vi "X-ray-images-mergening and calculating.vi"() -> ()   [LabVIEW 2019]
uses:
  <vilib>/Utility/file.llb/Write Delimited Spreadsheet (string).vi
  <vilib>/vision/NI_Vision_Development_Module.lvlib
  <vilib>/gmath/NI_Gmath.lvlib
  <vilib>/Analysis/NI_AALBase.lvlib
  imFillRemove_vs2019/x64/Release/imFillRemove_vs2019.dll
  distance_VS2019/x64/Release/distance_VS2019.dll
panel:
  out "Boolean":bool
  out "Path(part1)":path
  out "Path(part2)":path
  out "the lastest":string
  out "点击次数：":i32
  out "standard deviation 9":dbl format="%0.2f"
  out "mean 9":dbl format="%0.2f"
  out "standard deviation 8":dbl format="%0.2f"
  out "mean 8":dbl format="%0.2f"
  out "standard deviation 7":dbl format="%0.2f"
  out "mean 7":dbl format="%0.2f"
  out "standard deviation 6":dbl format="%0.2f"
  out "mean 6":dbl format="%0.2f"
  out "standard deviation 5":dbl format="%0.2f"
  out "mean 5":dbl format="%0.2f"
  out "Circularity":dbl[](array[numeric])
  out "Equivalent ellipse":dbl[](array[numeric])
  out "AR":dbl[](array[numeric])
  out "Perimeter":dbl[](array[numeric])
  out "Area":dbl[](array[numeric])
  out "耗时":u32
  out "属于某个角度下图像":T1(plugin-control)
  out "粒长":dbl[](array[numeric])
  out "粒宽":dbl[](array[numeric])
  out "长宽比":dbl[](array[numeric])
  out "mean 2":dbl format="%0.2f"
  out "standard deviation 2":dbl format="%0.2f"
  out "mean 3":dbl format="%0.2f"
  out "standard deviation 3":dbl format="%0.2f"
  out "mean 4":dbl format="%0.2f"
  out "standard deviation 4":dbl format="%0.2f"
  out "Number of Particles 2":i32
  out "单个粒子":T1(plugin-control)
  out "Combine Image final label 2":T1(plugin-control)
  in  "Removeareathreshold":i32=100
  in  "Range 2":cluster{"Lower value":sgl, "Upper value":sgl}={"Lower value"=1.0, "Upper value"=120.0}
  in  "数据存储":path=path "G:/preprocessing/rice_panicle/CT/data.xls"
  out "mean value 2":dbl
  in  "图片存储":path=path "G:/preprocessing/rice_panicle/CT/CT-merge"
  out "Combine Image":T1(plugin-control)
  out "Current Click Point":i32[](array[numeric])
  in  "CT images combine Stop":bool
  out "Click Points Array 2":i32[][](array[numeric])
  out "Combine Image final":T1(plugin-control)
  out "Combine Image final label":T1(plugin-control)
  out "Combine Image final label diatance":T1(plugin-control)
  out "Solid particle number（自动测量）":i32
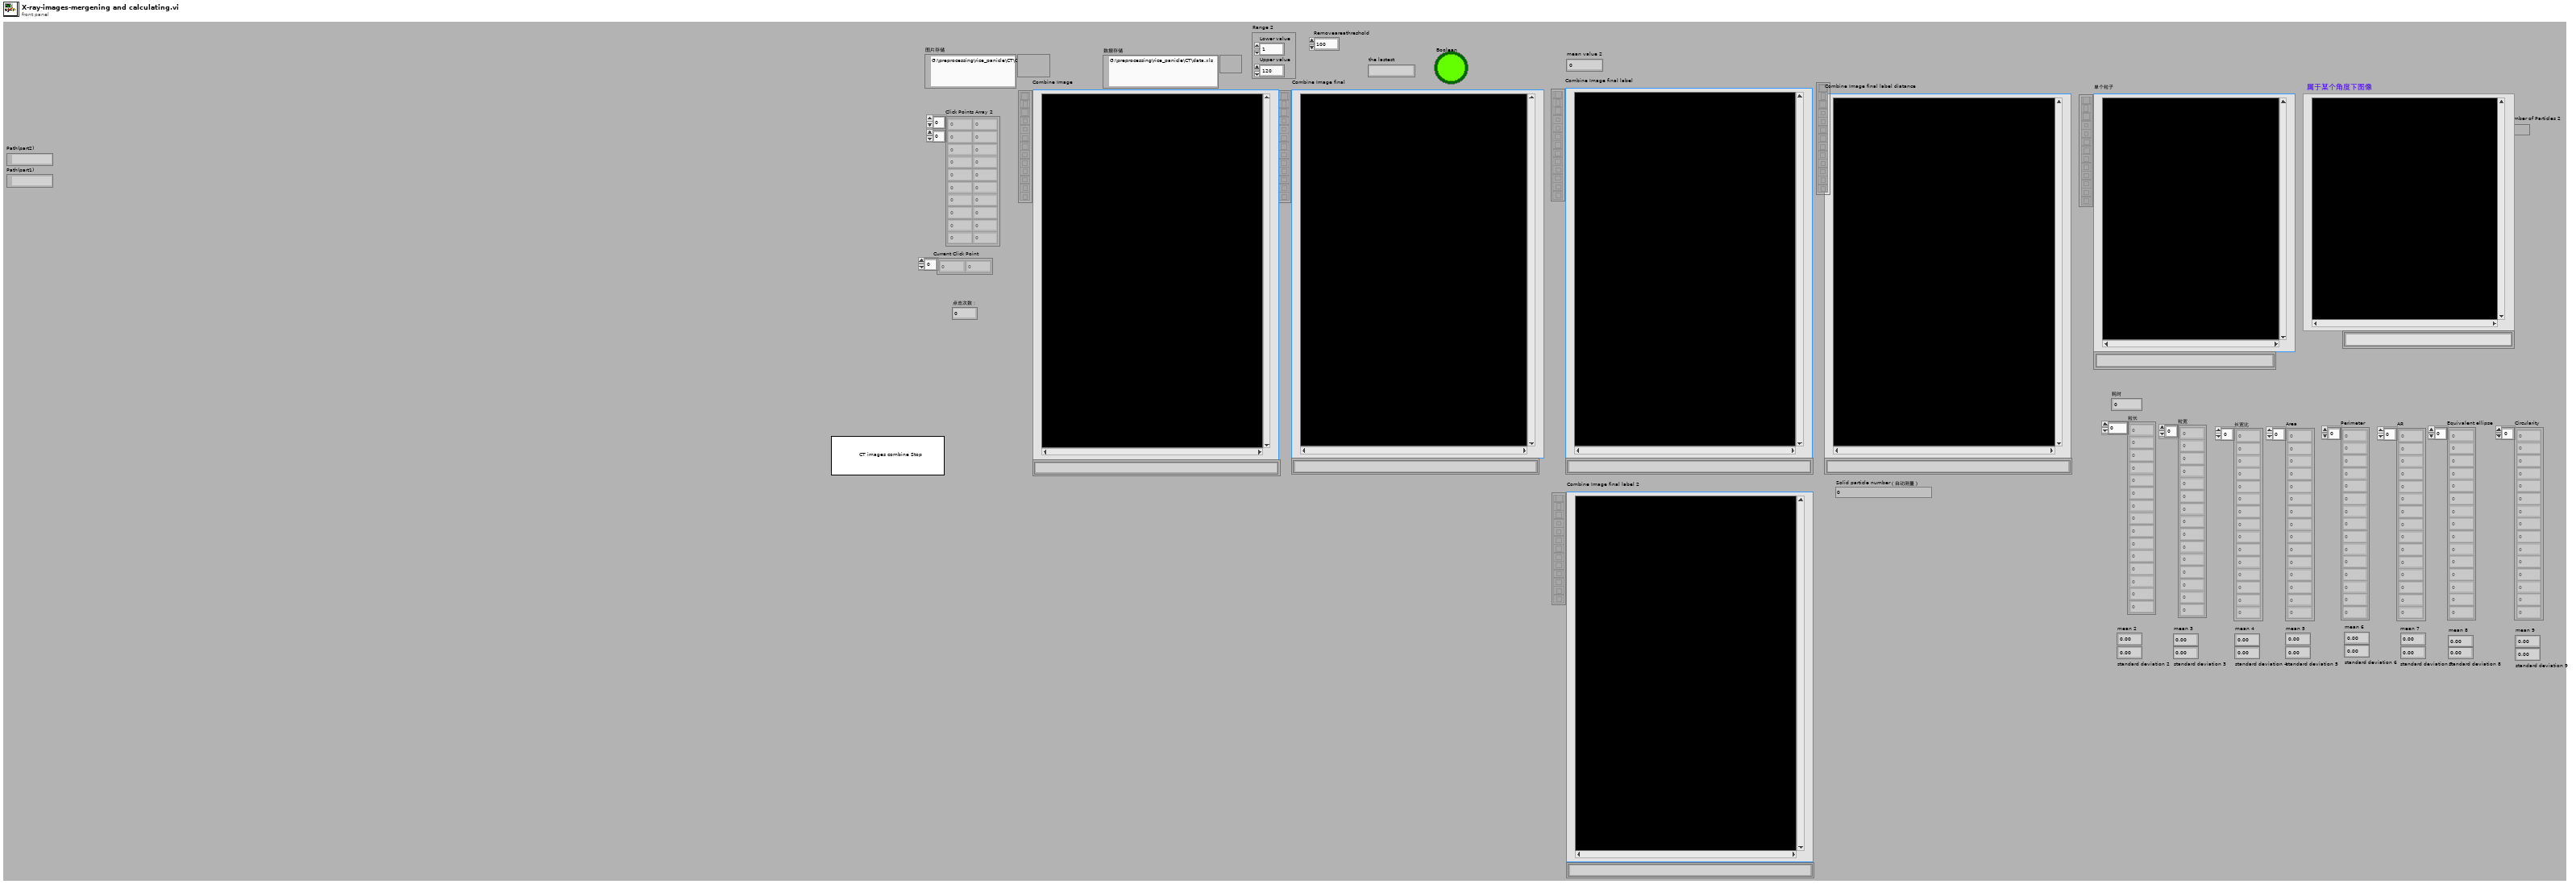
[diagram p1: front panel]
types:
  T1 = typedef "IMAQ Image.ctl" = refnum<image>
  T2 = typedef "Particle Parameters" = i32
  T3 = cluster{"Measurement Parameter":T2, "Range Lower Value":dbl, "Range Upper Value":dbl, "Range":bool, "Measurement Type":bool}
  T4 = enum16{"arithmetic", "geometric", "harmonic", "trimmed", "median"}
  T5 = typedef "Image Type" = u32
  T6 = cluster{"Measurement Parameter":T2, "Range Lower Value":dbl, "Range Upper Value":dbl, "Range":bool, "Measurement Type":bool}[]
  T7 = cluster{"Measurement Parameter":T2, dbl, dbl, "Range":bool, "Measurement Type":bool}
  T8 = cluster{"Measurement Parameter":T2, dbl, dbl, "Range":bool, "Measurement Type":bool}[]
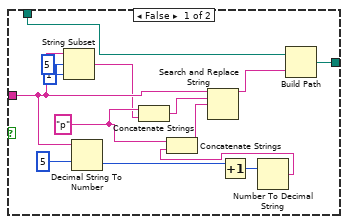
[diagram p2: hidden frame]
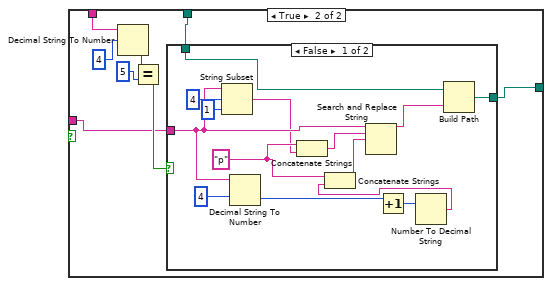
[diagram p3: hidden frame]
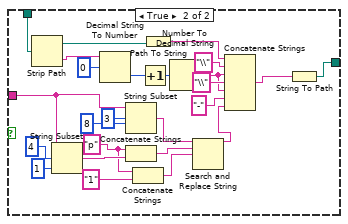
[diagram p4: hidden frame]
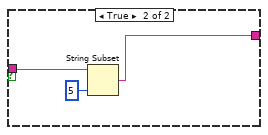
[diagram p5: hidden frame]
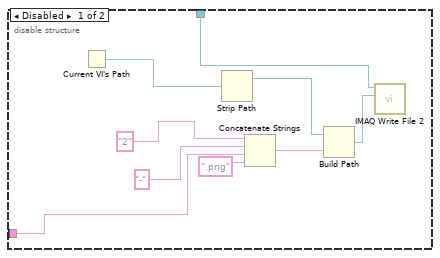
[diagram p6: hidden frame]
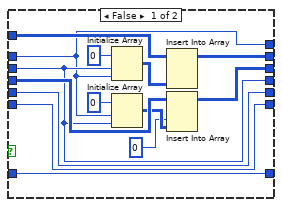
[diagram p8: hidden frame]
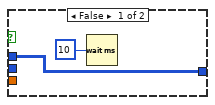
[diagram p9: hidden frame]
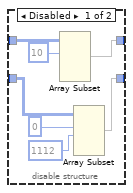
[diagram p10: hidden frame]
diagram:
  n1 = flat-sequence {
    tunnel: [w3] -> w2
    tunnel: [w5] -> w1
    frame #0 {
      n2 = call "IMAQ Load Image Dialog"("Prompt"="Select a panicle ct image (part1)") -> ("Path"=w3:path)  [unwired: 6 in, 4 out]
    }
    frame #1 {
      n3 = call "IMAQ Load Image Dialog"("Prompt"="Select a panicle ct image (part2)") -> ("Path"=w5:path)  [unwired: 6 in, 4 out]
    }
  }
  n4 = while {
    shift-right: [w12] -> _
    shift-left: w1 -> [w24]
    shift-right: [w11] -> _
    shift-left: w2 -> [w16]
    stop <- FALSE stop-if-true
    n5 = Strip Path(path=w16) -> (name=w18:string)  [unwired: 1 out]
    n6 = String Subset(string=w18, offset (0)=2, length (rest)=1 ("length (rest)")) -> (substring=w21:string)
    n7 = Equal?(x=w21, y="-") -> (x = y?=w19:bool)
    n8 = case shown="False" w19 {
      tunnel: w18 -> [w130 w133]
      tunnel: [w129 w132] -> w17
      frame False {
        n9 = String Subset(string=w130, length (rest)=6 ("length (rest)")) -> (substring=w129:string)  [unwired: 1 in]
      }
      frame True {
        n10 = String Subset(string=w133, length (rest)=5 ("length (rest)")) -> (substring=w132:string)  [unwired: 1 in]
      }
    }
    "the lastest" <- w17
    n11 = flat-sequence {
      tunnel: w16 -> [w136]
      tunnel: w24 -> [w135]
      frame #0 {
        w169 = T2[] [35, 19, 32, 50, 55] items=["Center of Mass X", "Center of Mass Y", "First Pixel X", "First Pixel Y", "Bounding Rect Left", "Bounding Rect Top", "Bounding Rect Right", "Bounding Rect Bottom", "Max Feret Diameter Start X", "Max Feret Diameter Start Y", "Max Feret Diameter End X", "Max Feret Diameter End Y", "Max Horiz. Segment Length Left", "Max Horiz. Segment Length Right", "Max Horiz. Segment Length Row", "-", "Bounding Rect Width", "Bounding Rect Height", "Bounding Rect Diagonal", "Perimeter", "Convex Hull Perimeter", "Holes' Perimeter", "Max Feret Diameter", "Equivalent Ellipse Major Axis", "Equivalent Ellipse Minor Axis", "Equivalent Ellipse Minor Axis (Feret)", "Equivalent Rect Long Side", "Equivalent Rect Short Side", "Equivalent Rect Diagonal", "Equivalent Rect Short Side (Feret)", "Average Horiz. Segment Length", "Average Vert. Segment Length", "Hydraulic Radius", "Waddel Disk Diameter", "-", "Area", "Holes' Area", "Particle & Holes' Area", "Convex Hull Area", "Image Area", "-", "Number of Holes", "Number of Horiz. Segments", "Number of Vert. Segments", "-", "Orientation", "Max Feret Diameter Orientation", "-", "% Area/Image Area", "% Area/(Particle & Holes' Area)", "Ratio of Equivalent Ellipse Axes", "Ratio of Equivalent Rect Sides", "-", "Elongation Factor", "Compactness Factor", "Heywood Circularity Factor", "Type Factor", "-", "Sum X", "Sum Y", "Sum XX", "Sum XY", "Sum YY", "Sum XXX", "Sum XXY", "Sum XYY", "Sum YYY", "-", "Moment of Inertia XX", "Moment of Inertia XY", "Moment of Inertia YY", "Moment of Inertia XXX", "Moment of Inertia XXY", "Moment of Inertia XYY", "Moment of Inertia YYY", "Norm. Moment of Inertia XX", "Norm. Moment of Inertia XY", "Norm. Moment of Inertia YY", "Norm. Moment of Inertia XXX", "Norm. Moment of Inertia XXY", "Norm. Moment of Inertia XYY", "Norm. Moment of Inertia YYY", "Hu Moment 1", "Hu Moment 2", "Hu Moment 3", "Hu Moment 4", "Hu Moment 5", "Hu Moment 6", "Hu Moment 7"] ("Pixel Measurements")
        w177 = T2[] [35] items=["Center of Mass X", "Center of Mass Y", "First Pixel X", "First Pixel Y", "Bounding Rect Left", "Bounding Rect Top", "Bounding Rect Right", "Bounding Rect Bottom", "Max Feret Diameter Start X", "Max Feret Diameter Start Y", "Max Feret Diameter End X", "Max Feret Diameter End Y", "Max Horiz. Segment Length Left", "Max Horiz. Segment Length Right", "Max Horiz. Segment Length Row", "-", "Bounding Rect Width", "Bounding Rect Height", "Bounding Rect Diagonal", "Perimeter", "Convex Hull Perimeter", "Holes' Perimeter", "Max Feret Diameter", "Equivalent Ellipse Major Axis", "Equivalent Ellipse Minor Axis", "Equivalent Ellipse Minor Axis (Feret)", "Equivalent Rect Long Side", "Equivalent Rect Short Side", "Equivalent Rect Diagonal", "Equivalent Rect Short Side (Feret)", "Average Horiz. Segment Length", "Average Vert. Segment Length", "Hydraulic Radius", "Waddel Disk Diameter", "-", "Area", "Holes' Area", "Particle & Holes' Area", "Convex Hull Area", "Image Area", "-", "Number of Holes", "Number of Horiz. Segments", "Number of Vert. Segments", "-", "Orientation", "Max Feret Diameter Orientation", "-", "% Area/Image Area", "% Area/(Particle & Holes' Area)", "Ratio of Equivalent Ellipse Axes", "Ratio of Equivalent Rect Sides", "-", "Elongation Factor", "Compactness Factor", "Heywood Circularity Factor", "Type Factor", "-", "Sum X", "Sum Y", "Sum XX", "Sum XY", "Sum YY", "Sum XXX", "Sum XXY", "Sum XYY", "Sum YYY", "-", "Moment of Inertia XX", "Moment of Inertia XY", "Moment of Inertia YY", "Moment of Inertia XXX", "Moment of Inertia XXY", "Moment of Inertia XYY", "Moment of Inertia YYY", "Norm. Moment of Inertia XX", "Norm. Moment of Inertia XY", "Norm. Moment of Inertia YY", "Norm. Moment of Inertia XXX", "Norm. Moment of Inertia XXY", "Norm. Moment of Inertia XYY", "Norm. Moment of Inertia YYY", "Hu Moment 1", "Hu Moment 2", "Hu Moment 3", "Hu Moment 4", "Hu Moment 5", "Hu Moment 6", "Hu Moment 7"] ("Pixel Measurements")
        w179 = T5 0 items=["Grayscale (U8)", "Grayscale (I16)", "Grayscale (SGL)", "Complex (CSG)", "RGB (U32)", "HSL (U32)", "RGB (U64)", "Grayscale (U16)"] ("Image Type")
        n12 = while {
          tunnel: [w435] -> _
          tunnel: [w434] -> w234
          tunnel: [w433] -> w232
          tunnel: [w432] -> w222
          tunnel: [w431] -> w221
          tunnel: w135 -> [w430]
          tunnel: [w429] -> w213
          tunnel: [w428] -> w207
          tunnel: [w419] -> w210
          tunnel: w136 -> [w418]
          stop <- w420 stop-if-true
          n13 = flat-sequence {
            tunnel: w430 -> [w444]
            tunnel: w418 -> [w446]
            tunnel: [w467] -> w427
            tunnel: [w464] -> w426
            tunnel: [w459] -> w425
            tunnel: [w456] -> w424
            tunnel: [w453] -> w423
            tunnel: [w445] -> w422
            tunnel: [w437] -> w421
            tunnel: [w444] -> w419
            tunnel: [w610] -> w428
            tunnel: [w611] -> w429
            tunnel: [w612] -> w431
            tunnel: [w613] -> w432
            tunnel: [w614] -> w433
            tunnel: [w615] -> w434
            tunnel: [w616] -> w435
            tunnel: w427 -> [w616]
            tunnel: w426 -> [w615]
            tunnel: w425 -> [w614]
            tunnel: w424 -> [w613]
            tunnel: w423 -> [w612]
            tunnel: w422 -> [w611]
            tunnel: w421 -> [w610]
            tunnel: [w609] -> w420
            frame #0 {
              w454 = u32 0 items=["Grayscale (U8)", "Grayscale (I16)", "Grayscale (SGL)", "Complex (CSG)", "RGB (U32)", "HSL (U32)", "RGB (U64)"] ("Image Type")
              w457 = u32 0 items=["Grayscale (U8)", "Grayscale (I16)", "Grayscale (SGL)", "Complex (CSG)", "RGB (U32)", "HSL (U32)", "RGB (U64)"] ("Image Type")
              w460 = u32 0 items=["Grayscale (U8)", "Grayscale (I16)", "Grayscale (SGL)", "Complex (CSG)", "RGB (U32)", "HSL (U32)", "RGB (U64)"] ("Image Type")
              w462 = u32 0 items=["Grayscale (U8)", "Grayscale (I16)", "Grayscale (SGL)", "Complex (CSG)", "RGB (U32)", "HSL (U32)", "RGB (U64)"] ("Image Type")
              w465 = u32 0 items=["Grayscale (U8)", "Grayscale (I16)", "Grayscale (SGL)", "Complex (CSG)", "RGB (U32)", "HSL (U32)", "RGB (U64)"] ("Image Type")
              w468 = u32 0 items=["Grayscale (U8)", "Grayscale (I16)", "Grayscale (SGL)", "Complex (CSG)", "RGB (U32)", "HSL (U32)", "RGB (U64)"] ("Image Type")
              w484 = u32 0 items=["Grayscale (U8)", "Grayscale (I16)", "Grayscale (SGL)", "Complex (CSG)", "RGB (U32)", "HSL (U32)", "RGB (U64)"] ("Image Type")
              w517 = i32[] [1] items=["No  event", "Click event", "Draw event", "Move event", "Size event", "Scroll event", "Activate event", "Close event", "Double click event"] ("Events list (all)")
              w528 = T5 0 items=["Grayscale (U8)", "Grayscale (I16)", "Grayscale (SGL)", "Complex (CSG)", "RGB (U32)", "HSL (U32)", "RGB (U64)", "Grayscale (U16)"] ("Image Type")
              w530 = T5 0 items=["Grayscale (U8)", "Grayscale (I16)", "Grayscale (SGL)", "Complex (CSG)", "RGB (U32)", "HSL (U32)", "RGB (U64)", "Grayscale (U16)"] ("Image Type")
              w537 = u32 0 items=["Grayscale (U8)", "Grayscale (I16)", "Grayscale (SGL)", "Complex (CSG)", "RGB (U32)", "HSL (U32)", "RGB (U64)"] ("Image Type")
              w540 = T5 0 items=["Grayscale (U8)", "Grayscale (I16)", "Grayscale (SGL)", "Complex (CSG)", "RGB (U32)", "HSL (U32)", "RGB (U64)", "Grayscale (U16)"] ("Image Type")
              w543 = T5 0 items=["Grayscale (U8)", "Grayscale (I16)", "Grayscale (SGL)", "Complex (CSG)", "RGB (U32)", "HSL (U32)", "RGB (U64)", "Grayscale (U16)"] ("Image Type")
              n14 = call "IMAQ Create"("Image Name"="part2", "Image Type"=w540) -> ("New Image"=w542:T1)  [unwired: 2 in, 2 out]
              n15 = call "IMAQ Create"("Image Name"="distance2_ct", "Image Type"=w457) -> ("New Image"=w456:T1)  [unwired: 2 in, 2 out]
              n16 = call "IMAQ Create"("Image Name"="part1", "Image Type"=w543) -> ("New Image"=w545:T1)  [unwired: 2 in, 2 out]
              n17 = call "IMAQ Create"("Image Name"="combine_final", "Image Type"=w484) -> ("New Image"=w483:T1)  [unwired: 2 in, 2 out]
              n18 = call "IMAQ Create"("Image Name"="part2 rotate", "Image Type"=w528) -> ("New Image"=w524:T1)  [unwired: 2 in, 2 out]
              n19 = call "IMAQ Create"("Image Name"="part1 rotate", "Image Type"=w530) -> ("New Image"=w526:T1)  [unwired: 2 in, 2 out]
              n20 = call "IMAQ Create"("Image Name"="combine", "Image Type"=w537) -> ("New Image"=w536:T1)  [unwired: 2 in, 2 out]
              n21 = call "IMAQ Create"("Image Name"="cluster_ct", "Image Type"=w462) -> ("New Image"=w445:T1)  [unwired: 2 in, 2 out]
              n22 = call "IMAQ Create"("Image Name"="threshold_ct", "Image Type"=w468) -> ("New Image"=w467:T1)  [unwired: 2 in, 2 out]
              n23 = call "IMAQ Create"("Image Name"="labelImage_ct", "Image Type"=w465) -> ("New Image"=w464:T1)  [unwired: 2 in, 2 out]
              n24 = call "IMAQ Create"("Image Name"="diatance_ct", "Image Type"=w460) -> ("New Image"=w459:T1)  [unwired: 2 in, 2 out]
              n25 = call "IMAQ Create"("Image Name"="labelImage3_ct", "Image Type"=w454) -> ("New Image"=w453:T1)  [unwired: 2 in, 2 out]
              n26 = call "IMAQ ReadFile"("File Path"=w444, "Image"=w542) -> ("Image Out"=w523:T1)  [unwired: 3 in, 6 out]
              n27 = call "IMAQ ReadFile"("File Path"=w446, "Image"=w545) -> ("Image Out"=w525:T1)  [unwired: 3 in, 6 out]
              n28 = call "IMAQ Rotate"("Maintain Size"=FALSE, "Angle (degrees)"=sgl 90.0, "Image Dst"=w524, "Image Src"=w523) -> ("Image Dst Out"=w531:T1)  [unwired: 4 in, 3 out]
              n29 = call "IMAQ Rotate"("Maintain Size"=FALSE, "Angle (degrees)"=sgl 90.0, "Image Dst"=w526, "Image Src"=w525) -> ("Image Dst Out"=w522:T1)  [unwired: 4 in, 3 out]
              n30 = call "IMAQ ImageToArray"("Image"=w531) -> ("Image Pixels (U8)"=w514:u8[][])  [unwired: 2 in, 5 out]
              n31 = call "IMAQ ImageToArray"("Image"=w522) -> ("Image Pixels (U8)"=w515:u8[][])  [unwired: 2 in, 5 out]
              n32 = disable-structure shown="Enabled" {
                disable-tunnel: w514 -> [w606 w607]
                disable-tunnel: w515 -> [w604 w608]
                disable-tunnel: [w601 w608] -> w521
                disable-tunnel: [w600 w607] -> w520
                frame Disabled {
                  n33 = Array Subset(array=w606, index (row)=10 ("index")) -> (w600:u8[][])  [unwired: 3 in]
                  n34 = Array Subset(array=w604, index (row)=0 ("index"), length (row)=1112 ("length")) -> (w601:u8[][])  [unwired: 2 in]
                }
                frame Enabled {
                }
              }
              n35 = Insert Into Array(array=w521, new element=w520) -> (w539:u8[][])  [unwired: 2 in]
              n36 = call "IMAQ ArrayToImage"("Image Pixels (U8)"=w539, "Image"=w536) -> ("Image Out"=w516:T1)  [unwired: 4 in, 5 out]
              "Combine Image" <- w516
              n37 = invoke on="Combine Image" class="ImageControl" method="Clear ROI"() -> (error out=w518:errorcluster)  [unwired: 3 in, 2 out]
              n38 = while {
                tunnel: w517 -> [w593]
                tunnel: w518 -> [_]
                shift-right: [w584] -> w506
                shift-left: i32[][] [] ("appended array") -> [w589]
                tunnel: w516 -> [_]
                tunnel: w515 -> [w588]
                tunnel: w514 -> [w587]
                tunnel: [w588] -> w500
                tunnel: [w587] -> w499
                stop <- w585 stop-if-true
                n39 = invoke on="Combine Image" class="ImageControl" method="Get Last Event"("Which Events"=w593) -> ("Type"=w592:i32, "Coordinates"=w591:i32[], "Other Parameters"=w590:sgl[])  [unwired: 7 in, 5 out]
                n40 = Not Equal To 0?(x=w592) -> (x != 0?=w594:bool)
                n41 = case shown="True" w594 {
                  tunnel: w591 -> [_ w598]
                  tunnel: w590 -> [_ _]
                  tunnel: w589 -> [w595 w599]
                  tunnel: [w595 w597] -> w584
                  frame False {
                    n42 = Wait (ms)(milliseconds to wait=u32 10) -> ()  [unwired: 1 out]
                  }
                  frame True {
                    n43 = Build Array (concatenate)(w599, w598) -> (w597:i32[][])
                    "Current Click Point" <- w598
                  }
                }
                n44 = Index Array(array=w584, index (col)=0 ("disabled index (col)")) -> (element=w582:i32[])  [unwired: 1 in]
                n45 = Array Size(array=w582) -> (size(s)=w581:i32)
                "点击次数：" <- w581
                n46 = Equal?(x=w581, y=2) -> (x = y?=w585:bool)
              }
              "Click Points Array 2" <- w506
              n47 = Array Size(array=w500) -> (size(s)=w496:i32[])
              n48 = Index Array(array=w506, index (row)=0) -> (element=w508:i32[])  [unwired: 1 in]
              n49 = Index Array(array=w506, index (row)=1) -> (element=w489:i32[])  [unwired: 1 in]
              n50 = Index Array(array=w496, index=1) -> (element=w494:i32)
              n51 = Index Array(array=w496, index=0) -> (element=w495:i32)
              n52 = Index Array(array=w508, index=1) -> (element=w498:i32)
              n53 = Index Array(array=w508, index=0) -> (element=w504:i32)
              n54 = Index Array(array=w489, index=0) -> (element=w503:i32)
              n55 = Index Array(array=w489, index=1) -> (element=w488:i32)
              n56 = Subtract(x=w504, y=w503) -> (x-y=w481:i32)
              n57 = Absolute Value(x=w481) -> (abs(x)=w482:i32)
              n58 = Greater Or Equal?(x=w481, y=0) -> (x >= y?=w501:bool)
              n59 = case shown="True" w501 {
                tunnel: w500 -> [w559 w568]
                tunnel: w499 -> [w556 w573]
                tunnel: w498 -> [w562 w577]
                tunnel: w495 -> [w563 w576]
                tunnel: w494 -> [w553 w570]
                tunnel: w482 -> [w554 w569]
                tunnel: [w560 w567] -> w493
                tunnel: [w555 w574] -> w492
                tunnel: [w562 w577] -> w491
                tunnel: [w563 w576] -> w478
                tunnel: w488 -> [w561 w575]
                tunnel: [w561 w575] -> w480
                tunnel: [w553 w570] -> _
                tunnel: [w554 w569] -> w476
                frame False {
                  n60 = Initialize Array(u8 0 ("element"), w554, w553) -> (w565:u8[][])
                  n61 = Initialize Array(u8 0 ("element"), w553, w554) -> (w558:u8[][])
                  n62 = Insert Into Array(array=w556, new element=w565) -> (w555:u8[][])  [unwired: 2 in]
                  n63 = Insert Into Array(array=w559, index (col)=0 ("disabled index (col)"), new element=w558) -> (w560:u8[][])  [unwired: 1 in]
                }
                frame True {
                  n64 = Initialize Array(u8 0 ("element"), w570, w569) -> (w571:u8[][])
                  n65 = Initialize Array(u8 0 ("element"), w570, w569) -> (w579:u8[][])
                  n66 = Insert Into Array(array=w573, index (col)=0 ("disabled index (col)"), new element=w571) -> (w574:u8[][])  [unwired: 1 in]
                  n67 = Insert Into Array(array=w568, new element=w579) -> (w567:u8[][])  [unwired: 2 in]
                }
              }
              n68 = Subtract(x=w480, y=w478) -> (x-y=w479:i32)
              n69 = Array Subset(array=w493, index (row)=0 ("index"), length (row)=w491) -> (w487:u8[][])  [unwired: 2 in]
              n70 = Add(x=w476, y=10) -> (x+y=w475:i32)
              n71 = Array Subset(array=w492, index (row)=w479) -> (w486:u8[][])  [unwired: 3 in]
              n72 = Insert Into Array(array=w487, new element=w486) -> (w473:u8[][])  [unwired: 2 in]
              n73 = Array Subset(array=w473, index (row)=10 ("index"), length (row)=2600 ("length"), index (col)=w475, length (col)=1850 ("length")) -> (w470:u8[][])
              n74 = call "IMAQ ArrayToImage"("Image Pixels (U8)"=w470, "Image"=w483) -> ("Image Out"=w447:T1)  [unwired: 4 in, 5 out]
              n75 = call "IMAQ ImageBorderSize"("Get/Set Status? (Set)"=TRUE, "Image"=w447, "Image border size in"=5 ("Border Size")) -> ("Image Out"=w449:T1)  [unwired: 1 in, 2 out]
              n76 = call "IMAQ Convolute"("Kernel"=sgl[][] [[1.0, 2.0, 1.0], [2.0, 4.0, 2.0], [1.0, 2.0, 1.0]], "Divider (kernel sum)"=sgl 0.0 ("Divider"), "Image Src"=w449) -> ("Image Dst Out"=w436:T1)  [unwired: 4 in, 4 out]
              n77 = call "IMAQ GetImageSize"("Image"=w436) -> ("Y Resolution"=w443:i32, "X Resolution"=w438:i32)  [unwired: 3 in, 1 out]
              n78 = while {
                tunnel: w436 -> [w552]
                shift-right: [w548] -> _
                shift-left: w443 -> [w549]
                tunnel: [w548] -> w440
                stop <- w550 stop-if-true
                n79 = Decrement(x=w549) -> (x-1=w548:i32)
                n80 = call "IMAQ GetPixelValue"("Image"=w552, "X Coordinate"=0, "Y Coordinate"=w548) -> ("Pixel Value (I16)"=w547:i16)  [unwired: 3 in, 4 out]
                n81 = Greater Or Equal?(x=w547, y=i16 50) -> (x >= y?=w550:bool)
              }
              n82 = Build Array(0, 0, w438, w440) -> (w439:i32[])
              n83 = call "IMAQ Extract 2"("Optional Rectangle"=w439, "Image Src"=w436) -> ("Image Dst Out"=w437:T1)  [unwired: 8 in, 1 out]
              "Combine Image final" <- w437
            }
            frame #1 {
              n84 = call "Prompt User for Input"() -> ("OK"=w609:bool)  [unwired: 2 in, 17 out]
            }
          }
        }
        n85 = Unbundle By Name("Range 2") -> ("Lower value"=w189:sgl, "Upper value"=w188:sgl)
        n86 = while {
          tunnel: w234 -> [w362]
          tunnel: [w361] -> w224
          tunnel: w213 -> [w360]
          tunnel: w207 -> [w358]
          tunnel: [w359] -> w212
          shift-right: [w354] -> _
          shift-left: w189 -> [w349]
          shift-right: [w353] -> _
          shift-left: w188 -> [w347]
          tunnel: "Range 2" -> [w351]
          tunnel: [w346] -> w186
          tunnel: [w345] -> w155
          stop <- w355 stop-if-true
          n87 = Bundle By Name(cluster=w351, "Lower value"=w349, "Upper value"=w347) -> (w352:cluster{"Lower value":sgl, "Upper value":sgl})
          n88 = flat-sequence {
            tunnel: w362 -> [w406]
            tunnel: w360 -> [w404]
            tunnel: w358 -> [w402]
            tunnel: [w405] -> w357
            tunnel: [w403] -> w356
            tunnel: w352 -> [w374]
            tunnel: [w373] -> w350
            tunnel: w349 -> [w373]
            tunnel: [w372] -> w348
            tunnel: w347 -> [w372]
            tunnel: [w367] -> w346
            tunnel: [w363] -> w345
            tunnel: [w412] -> w359
            tunnel: [w413] -> w361
            tunnel: w357 -> [w413]
            tunnel: w356 -> [w412]
            tunnel: [w407] -> w355
            tunnel: [w411] -> w354
            tunnel: [w410] -> w353
            tunnel: w350 -> [w409]
            tunnel: w348 -> [w408]
            frame #0 {
              w370 = T5 0 items=["Grayscale (U8)", "Grayscale (I16)", "Grayscale (SGL)", "Complex (CSG)", "RGB (U32)", "HSL (U32)", "RGB (U64)", "Grayscale (U16)"] ("Image Type")
              w379 = T5 0 items=["Grayscale (U8)", "Grayscale (I16)", "Grayscale (SGL)", "Complex (CSG)", "RGB (U32)", "HSL (U32)", "RGB (U64)", "Grayscale (U16)"] ("Image Type")
              w392 = T2[] [35] items=["Center of Mass X", "Center of Mass Y", "First Pixel X", "First Pixel Y", "Bounding Rect Left", "Bounding Rect Top", "Bounding Rect Right", "Bounding Rect Bottom", "Max Feret Diameter Start X", "Max Feret Diameter Start Y", "Max Feret Diameter End X", "Max Feret Diameter End Y", "Max Horiz. Segment Length Left", "Max Horiz. Segment Length Right", "Max Horiz. Segment Length Row", "-", "Bounding Rect Width", "Bounding Rect Height", "Bounding Rect Diagonal", "Perimeter", "Convex Hull Perimeter", "Holes' Perimeter", "Max Feret Diameter", "Equivalent Ellipse Major Axis", "Equivalent Ellipse Minor Axis", "Equivalent Ellipse Minor Axis (Feret)", "Equivalent Rect Long Side", "Equivalent Rect Short Side", "Equivalent Rect Diagonal", "Equivalent Rect Short Side (Feret)", "Average Horiz. Segment Length", "Average Vert. Segment Length", "Hydraulic Radius", "Waddel Disk Diameter", "-", "Area", "Holes' Area", "Particle & Holes' Area", "Convex Hull Area", "Image Area", "-", "Number of Holes", "Number of Horiz. Segments", "Number of Vert. Segments", "-", "Orientation", "Max Feret Diameter Orientation", "-", "% Area/Image Area", "% Area/(Particle & Holes' Area)", "Ratio of Equivalent Ellipse Axes", "Ratio of Equivalent Rect Sides", "-", "Elongation Factor", "Compactness Factor", "Heywood Circularity Factor", "Type Factor", "-", "Sum X", "Sum Y", "Sum XX", "Sum XY", "Sum YY", "Sum XXX", "Sum XXY", "Sum XYY", "Sum YYY", "-", "Moment of Inertia XX", "Moment of Inertia XY", "Moment of Inertia YY", "Moment of Inertia XXX", "Moment of Inertia XXY", "Moment of Inertia XYY", "Moment of Inertia YYY", "Norm. Moment of Inertia XX", "Norm. Moment of Inertia XY", "Norm. Moment of Inertia YY", "Norm. Moment of Inertia XXX", "Norm. Moment of Inertia XXY", "Norm. Moment of Inertia XYY", "Norm. Moment of Inertia YYY", "Hu Moment 1", "Hu Moment 2", "Hu Moment 3", "Hu Moment 4", "Hu Moment 5", "Hu Moment 6", "Hu Moment 7"] ("Pixel Measurements")
              w399 = T5 0 items=["Grayscale (U8)", "Grayscale (I16)", "Grayscale (SGL)", "Complex (CSG)", "RGB (U32)", "HSL (U32)", "RGB (U64)", "Grayscale (U16)"] ("Image Type")
              # "去除小区域"
              # "直接用总面积/平均面积"
              # "去除小区域"
              n89 = call "IMAQ Threshold"("Range"=w374, "Image Dst"=w404, "Image Src"=w402) -> ("Image Dst Out"=w393:T1)  [unwired: 3 in, 5 out]
              n90 = call "IMAQ ImageToArray"("Image"=w393) -> ("Image Pixels (U8)"=w394:u8[][])  [unwired: 2 in, 5 out]
              n91 = call "IMAQ GetImageSize"("Image"=w393) -> ("Y Resolution"=w396:i32, "X Resolution"=w395:i32)  [unwired: 1 in, 3 out]
              n92 = call "IMAQ Create"("Image Name"="BW_color4", "Image Type"=w399) -> ("New Image"=w397:T1)  [unwired: 2 in, 2 out]
              n93 = dll-call lib="G:/preprocessing/rice_panicle/imFillRemove_vs2019/x64/Release/imFillRemove_vs2019.dll" fn="bwremove"("bw"=w394, "row"=w396, "col"=w395, "areathreshold"="Removeareathreshold") -> ("bw"=w401:u8[][])  [unwired: 6 in, 3 out]
              n94 = call "IMAQ ArrayToImage"("Image Pixels (U8)"=w401, "Image"=w397) -> ("Image Out"=w377:T1)  [unwired: 4 in, 5 out]
              n95 = call "IMAQ Particle Analysis"("Pixel Measurements"=w392, "Image"=w377) -> ("Particle Measurements (Pixels)"=w387:dbl[][])  [unwired: 3 in, 6 out]
              n96 = Index Array(array=w387, index (col)=0 ("index (row)")) -> (element=w390:dbl[])  [unwired: 1 in]
              n97 = call <vilib>:"Measures of Mean.vi"("percent (trim)"=25.0, "type"=T4."trimmed", "x array"=w390) -> ("mean value"=w386:dbl)  [unwired: 8 out]
              "mean value 2" <- w386
              n98 = Divide(x=w386, y=3.0) -> (x/y=w376:dbl)
              n99 = call "IMAQ ImageToArray"("Image"=w377) -> ("Image Pixels (U8)"=w384:u8[][])  [unwired: 2 in, 5 out]
              n100 = call "IMAQ GetImageSize"("Image"=w377) -> ("Y Resolution"=w382:i32, "X Resolution"=w383:i32)  [unwired: 1 in, 3 out]
              n101 = To Long Integer(number=w376) -> (32bit integer=w375:i32)
              n102 = call "IMAQ Create"("Image Name"="BW_color5", "Image Type"=w379) -> ("New Image"=w381:T1)  [unwired: 2 in, 2 out]
              n103 = dll-call lib="G:/preprocessing/rice_panicle/imFillRemove_vs2019/x64/Release/imFillRemove_vs2019.dll" fn="bwremove"("bw"=w384, "row"=w382, "col"=w383, "areathreshold"=w375) -> ("bw"=w378:u8[][])  [unwired: 6 in, 3 out]
              n104 = call "IMAQ ArrayToImage"("Image Pixels (U8)"=w378, "Image"=w381) -> ("Image Out"=w364:T1)  [unwired: 4 in, 5 out]
              n105 = call <vilib>:"IVA GrayFilters - NthOrder.vi"("Filter size Y"=3, "Filter size X"=3, "Image In"=w364) -> ("Image Out"=w363:T1)  [unwired: 1 in, 7 out]
              n106 = call "IMAQ Label"("Image Dst"=w406, "Image Src"=w363) -> ("Number of Particles"=w405:i32, "Image Dst Out"=w403:T1)  [unwired: 2 in, 1 out]
              "Combine Image final label" <- w403
              n107 = call "IMAQ Create"("Image Name"="BW_color3", "Image Type"=w370) -> ("New Image"=w368:T1)  [unwired: 2 in, 2 out]
              n108 = call "IMAQ Multiply"("Image Src A"=w363, "Constant"=255.0, "Image Dst"=w368) -> ("Image Dst Out"=w367:T1)  [unwired: 4 in, 1 out]
              "Combine Image final label 2" <- w367
            }
            frame #1 {
              n109 = call "Prompt User for Input2"() -> ("OK"=w407:bool)  [unwired: 2 in, 17 out]
              n110 = case shown="False" w407 {
                tunnel: [w415 w417] -> w411
                tunnel: [w414 w416] -> w410
                tunnel: w409 -> [_ w417]
                tunnel: w408 -> [_ w416]
                frame False {
                  n111 = call "Prompt User for Input3"() -> ("Upper value"=w414:dbl, "Lower value"=w415:dbl)  [unwired: 2 in, 16 out]
                }
                frame True {
                }
              }
              n112 = local write "Boolean"(w407) -> ()
            }
          }
        }
        n113 = Strip Path(path=w210) -> (name=w196:string)  [unwired: 1 out]
        n114 = String Length(string=w196) -> (length=w199:i32)
        n115 = Subtract(x=w199, y=6) -> (x-y=w197:i32)
        n116 = String Subset(string=w196, offset (0)=0, length (rest)=w197) -> (substring=w195:string)
        n117 = Concatenate Strings(w195, "-original" ("string"), ".png" ("string")) -> (w209:string)
        n118 = Build Path(base path="图片存储", name or relative path=w209) -> (appended path=w208:path)
        n119 = call-poly "IMAQ Write File 2"("File Path"=w208, "Image"=w207) -> ()  [unwired: 4 in, 6 out]
        n120 = Concatenate Strings(w195, "-preprocessing" ("string"), ".png" ("string")) -> (w201:string)
        n121 = call "IMAQ Distance"("Image Dst"=w232, "Image Src"=w212, "Square/Hexa (Square)"=FALSE) -> ("Image Dst Out"=w225:T1)  [unwired: 1 in, 3 out]
        n122 = Build Path(base path="图片存储", name or relative path=w201) -> (appended path=w202:path)
        n123 = call "IMAQ ImageToArray"("Image"=w212) -> ("Image Pixels (U8)"=w230:u8[][])  [unwired: 2 in, 5 out]
        n124 = call "IMAQ GetImageSize"("Image"=w212) -> ("Y Resolution"=w229:i32, "X Resolution"=w228:i32)  [unwired: 1 in, 3 out]
        n125 = call-poly "IMAQ Write File 2"("File Path"=w202, "Image"=w186) -> ()  [unwired: 4 in, 6 out]
        n126 = call "IMAQ ImageToArray"("Image"=w225) -> ("Image Pixels (U8)"=w226:u8[][])  [unwired: 2 in, 5 out]
        n127 = Initialize Array(u8 0 ("element"), w229, w228) -> (w227:u8[][])
        n128 = dll-call lib="G:/preprocessing/rice_panicle/distance_VS2019/x64/Release/distance_VS2019.dll" fn="distance"("imageData1"=w230, "imageData2"=w226, "widrh"=w229, "height"=w228, "numberoflabel"=w224, "resultImage"=w227) -> ("resultImage"=w223:u8[][])  [unwired: 8 in, 3 out]
        n129 = call "IMAQ ArrayToImage"("Image Pixels (U8)"=w223, "Image"=w222) -> ("Image Out"=w215:T1)  [unwired: 4 in, 5 out]
        n130 = call "IMAQ RemoveParticle"("Connectivity 4/8 (8)"=TRUE, "Low Pass/High Pass (Low)"=FALSE, "Square/Hexa (Square)"=FALSE, "Number of Erosion"=1, "Image Src"=w215) -> ("Image Dst Out"=w214:T1)  [unwired: 2 in, 4 out]
        n131 = call "IMAQ Label"("Image Dst"=w221, "Image Src"=w214) -> ("Number of Particles"=w194:i32, "Image Dst Out"=→"Combine Image final label diatance":T1)  [unwired: 2 in, 1 out]
        "Solid particle number（自动测量）" <- w194
        n132 = call "IMAQ Particle Analysis"("Pixel Measurements"=w177, "Image"=w155) -> ("Particle Measurements (Pixels)"=w175:dbl[][])  [unwired: 3 in, 6 out]
        n133 = Index Array(array=w175, index (col)=0 ("index (row)")) -> (element=w174:dbl[])  [unwired: 1 in]
        n134 = call <vilib>:"Std Deviation and Variance.vi"("X"=w174) -> ("mean"=w173:dbl, "standard deviation"=w172:dbl)  [unwired: 1 in, 1 out]
        n135 = Subtract(x=w173, y=w172) -> (x-y=w171:dbl)
        n136 = Add(x=w173, y=w172) -> (x+y=w170:dbl)
        n137 = Bundle(cluster=T3 {"Measurement Parameter"=35, "Range Lower Value"=0.0, "Range Upper Value"=0.0, "Range"=FALSE, "Measurement Type"=FALSE} ("Selection Value"), "Range Lower Value"=w171, "Range Upper Value"=w170) -> (w183:T3)  [unwired: 3 out]
        n138 = Initialize Array(w183, 1 ("dimension size")) -> (w184:T6)
        n139 = call "IMAQ Create"("Image Name"="S2", "Image Type"=w179) -> ("New Image"=w181:T1)  [unwired: 2 in, 2 out]
        n140 = call "IMAQ Particle Filter 3"("Image Src"=w155, "Image Dst"=w181, "Selection Values"=w184, "Keep/Remove Particles (F)"=FALSE) -> ("Image Dst Out"=w167:T1, "Number of Particles"=w166:i32)  [unwired: 5 in, 5 out]
        "单个粒子" <- w167
        "Number of Particles 2" <- w166
        n141 = flat-sequence {
          tunnel: w166 -> [w246]
          tunnel: w167 -> [w247]
          tunnel: [w247] -> w244
          tunnel: [w246] -> w243
          tunnel: [w245] -> w242
          tunnel: w244 -> [w263]
          tunnel: w243 -> [w262]
          tunnel: w242 -> [w261]
          tunnel: [w261] -> w241
          tunnel: [w253] -> w240
          tunnel: [w252] -> w239
          tunnel: [w251] -> w238
          tunnel: [w250] -> w237
          tunnel: [w249] -> w236
          tunnel: [w248] -> w235
          tunnel: w241 -> [w343]
          tunnel: [w341] -> w154
          tunnel: w240 -> [w341]
          tunnel: [w340] -> w153
          tunnel: w239 -> [w340]
          tunnel: [w339] -> w152
          tunnel: w238 -> [w339]
          tunnel: [w338] -> w151
          tunnel: w237 -> [w338]
          tunnel: [w337] -> w150
          tunnel: w236 -> [w337]
          tunnel: [w336] -> w149
          tunnel: w235 -> [w336]
          frame #0 {
            n142 = Tick Count (ms)() -> (millisecond timer value=w245:u32)
          }
          frame #1 {
            w272 = T2[] [0, 1, 45] items=["Center of Mass X", "Center of Mass Y", "First Pixel X", "First Pixel Y", "Bounding Rect Left", "Bounding Rect Top", "Bounding Rect Right", "Bounding Rect Bottom", "Max Feret Diameter Start X", "Max Feret Diameter Start Y", "Max Feret Diameter End X", "Max Feret Diameter End Y", "Max Horiz. Segment Length Left", "Max Horiz. Segment Length Right", "Max Horiz. Segment Length Row", "-", "Bounding Rect Width", "Bounding Rect Height", "Bounding Rect Diagonal", "Perimeter", "Convex Hull Perimeter", "Holes' Perimeter", "Max Feret Diameter", "Equivalent Ellipse Major Axis", "Equivalent Ellipse Minor Axis", "Equivalent Ellipse Minor Axis (Feret)", "Equivalent Rect Long Side", "Equivalent Rect Short Side", "Equivalent Rect Diagonal", "Equivalent Rect Short Side (Feret)", "Average Horiz. Segment Length", "Average Vert. Segment Length", "Hydraulic Radius", "Waddel Disk Diameter", "-", "Area", "Holes' Area", "Particle & Holes' Area", "Convex Hull Area", "Image Area", "-", "Number of Holes", "Number of Horiz. Segments", "Number of Vert. Segments", "-", "Orientation", "Max Feret Diameter Orientation", "-", "% Area/Image Area", "% Area/(Particle & Holes' Area)", "Ratio of Equivalent Ellipse Axes", "Ratio of Equivalent Rect Sides", "-", "Elongation Factor", "Compactness Factor", "Heywood Circularity Factor", "Type Factor", "-", "Sum X", "Sum Y", "Sum XX", "Sum XY", "Sum YY", "Sum XXX", "Sum XXY", "Sum XYY", "Sum YYY", "-", "Moment of Inertia XX", "Moment of Inertia XY", "Moment of Inertia YY", "Moment of Inertia XXX", "Moment of Inertia XXY", "Moment of Inertia XYY", "Moment of Inertia YYY", "Norm. Moment of Inertia XX", "Norm. Moment of Inertia XY", "Norm. Moment of Inertia YY", "Norm. Moment of Inertia XXX", "Norm. Moment of Inertia XXY", "Norm. Moment of Inertia XYY", "Norm. Moment of Inertia YYY", "Hu Moment 1", "Hu Moment 2", "Hu Moment 3", "Hu Moment 4", "Hu Moment 5", "Hu Moment 6", "Hu Moment 7"] ("Pixel Measurements")
            # "粒宽"
            # "粒长"
            n143 = call "IMAQ Particle Analysis"("Pixel Measurements"=w272, "Image"=w263) -> ("Particle Measurements (Pixels)"=w270:dbl[][], "Image Out (duplicate)"=w271:T1)  [unwired: 3 in, 5 out]
            n144 = Index Array(array=w270, index (col) #1=0 ("disabled index (col)"), index (col) #2=1 ("index (col)"), index (col) #3=2 ("index (col)")) -> (element #1=w266:dbl[], element #2=w265:dbl[], element #3=w264:dbl[])  [unwired: 3 in]
            n145 = for {
              N: w262 -> [_]
              tunnel: w271 -> [w324]
              tunnel: w266 -> [w301] mode=indexing
              tunnel: w265 -> [w295] mode=indexing
              tunnel: w264 -> [w316] mode=indexing
              tunnel: [w307] -> _ mode=indexing
              tunnel: [w284] -> w257 mode=indexing
              tunnel: [w281] -> w258 mode=indexing
              i -> [w313]
              w282 = T2[] [17] items=["Center of Mass X", "Center of Mass Y", "First Pixel X", "First Pixel Y", "Bounding Rect Left", "Bounding Rect Top", "Bounding Rect Right", "Bounding Rect Bottom", "Max Feret Diameter Start X", "Max Feret Diameter Start Y", "Max Feret Diameter End X", "Max Feret Diameter End Y", "Max Horiz. Segment Length Left", "Max Horiz. Segment Length Right", "Max Horiz. Segment Length Row", "-", "Bounding Rect Width", "Bounding Rect Height", "Bounding Rect Diagonal", "Perimeter", "Convex Hull Perimeter", "Holes' Perimeter", "Max Feret Diameter", "Equivalent Ellipse Major Axis", "Equivalent Ellipse Minor Axis", "Equivalent Ellipse Minor Axis (Feret)", "Equivalent Rect Long Side", "Equivalent Rect Short Side", "Equivalent Rect Diagonal", "Equivalent Rect Short Side (Feret)", "Average Horiz. Segment Length", "Average Vert. Segment Length", "Hydraulic Radius", "Waddel Disk Diameter", "-", "Area", "Holes' Area", "Particle & Holes' Area", "Convex Hull Area", "Image Area", "-", "Number of Holes", "Number of Horiz. Segments", "Number of Vert. Segments", "-", "Orientation", "Max Feret Diameter Orientation", "-", "% Area/Image Area", "% Area/(Particle & Holes' Area)", "Ratio of Equivalent Ellipse Axes", "Ratio of Equivalent Rect Sides", "-", "Elongation Factor", "Compactness Factor", "Heywood Circularity Factor", "Type Factor", "-", "Sum X", "Sum Y", "Sum XX", "Sum XY", "Sum YY", "Sum XXX", "Sum XXY", "Sum XYY", "Sum YYY", "-", "Moment of Inertia XX", "Moment of Inertia XY", "Moment of Inertia YY", "Moment of Inertia XXX", "Moment of Inertia XXY", "Moment of Inertia XYY", "Moment of Inertia YYY", "Norm. Moment of Inertia XX", "Norm. Moment of Inertia XY", "Norm. Moment of Inertia YY", "Norm. Moment of Inertia XXX", "Norm. Moment of Inertia XXY", "Norm. Moment of Inertia XYY", "Norm. Moment of Inertia YYY", "Hu Moment 1", "Hu Moment 2", "Hu Moment 3", "Hu Moment 4", "Hu Moment 5", "Hu Moment 6", "Hu Moment 7"] ("Pixel Measurements")
              w287 = T2[] [16] items=["Center of Mass X", "Center of Mass Y", "First Pixel X", "First Pixel Y", "Bounding Rect Left", "Bounding Rect Top", "Bounding Rect Right", "Bounding Rect Bottom", "Max Feret Diameter Start X", "Max Feret Diameter Start Y", "Max Feret Diameter End X", "Max Feret Diameter End Y", "Max Horiz. Segment Length Left", "Max Horiz. Segment Length Right", "Max Horiz. Segment Length Row", "-", "Bounding Rect Width", "Bounding Rect Height", "Bounding Rect Diagonal", "Perimeter", "Convex Hull Perimeter", "Holes' Perimeter", "Max Feret Diameter", "Equivalent Ellipse Major Axis", "Equivalent Ellipse Minor Axis", "Equivalent Ellipse Minor Axis (Feret)", "Equivalent Rect Long Side", "Equivalent Rect Short Side", "Equivalent Rect Diagonal", "Equivalent Rect Short Side (Feret)", "Average Horiz. Segment Length", "Average Vert. Segment Length", "Hydraulic Radius", "Waddel Disk Diameter", "-", "Area", "Holes' Area", "Particle & Holes' Area", "Convex Hull Area", "Image Area", "-", "Number of Holes", "Number of Horiz. Segments", "Number of Vert. Segments", "-", "Orientation", "Max Feret Diameter Orientation", "-", "% Area/Image Area", "% Area/(Particle & Holes' Area)", "Ratio of Equivalent Ellipse Axes", "Ratio of Equivalent Rect Sides", "-", "Elongation Factor", "Compactness Factor", "Heywood Circularity Factor", "Type Factor", "-", "Sum X", "Sum Y", "Sum XX", "Sum XY", "Sum YY", "Sum XXX", "Sum XXY", "Sum XYY", "Sum YYY", "-", "Moment of Inertia XX", "Moment of Inertia XY", "Moment of Inertia YY", "Moment of Inertia XXX", "Moment of Inertia XXY", "Moment of Inertia XYY", "Moment of Inertia YYY", "Norm. Moment of Inertia XX", "Norm. Moment of Inertia XY", "Norm. Moment of Inertia YY", "Norm. Moment of Inertia XXX", "Norm. Moment of Inertia XXY", "Norm. Moment of Inertia XYY", "Norm. Moment of Inertia YYY", "Hu Moment 1", "Hu Moment 2", "Hu Moment 3", "Hu Moment 4", "Hu Moment 5", "Hu Moment 6", "Hu Moment 7"] ("Pixel Measurements")
              w290 = T5 0 items=["Grayscale (U8)", "Grayscale (I16)", "Grayscale (SGL)", "Complex (CSG)", "RGB (U32)", "HSL (U32)", "RGB (U64)", "Grayscale (U16)"] ("Image Type")
              w303 = T5 0 items=["Grayscale (U8)", "Grayscale (I16)", "Grayscale (SGL)", "Complex (CSG)", "RGB (U32)", "HSL (U32)", "RGB (U64)", "Grayscale (U16)"] ("Image Type")
              w320 = T2 1 items=["Center of Mass X", "Center of Mass Y", "First Pixel X", "First Pixel Y", "Bounding Rect Left", "Bounding Rect Top", "Bounding Rect Right", "Bounding Rect Bottom", "Max Feret Diameter Start X", "Max Feret Diameter Start Y", "Max Feret Diameter End X", "Max Feret Diameter End Y", "Max Horiz. Segment Length Left", "Max Horiz. Segment Length Right", "Max Horiz. Segment Length Row", "-", "Bounding Rect Width", "Bounding Rect Height", "Bounding Rect Diagonal", "Perimeter", "Convex Hull Perimeter", "Holes' Perimeter", "Max Feret Diameter", "Equivalent Ellipse Major Axis", "Equivalent Ellipse Minor Axis", "Equivalent Ellipse Minor Axis (Feret)", "Equivalent Rect Long Side", "Equivalent Rect Short Side", "Equivalent Rect Diagonal", "Equivalent Rect Short Side (Feret)", "Average Horiz. Segment Length", "Average Vert. Segment Length", "Hydraulic Radius", "Waddel Disk Diameter", "-", "Area", "Holes' Area", "Particle & Holes' Area", "Convex Hull Area", "Image Area", "-", "Number of Holes", "Number of Horiz. Segments", "Number of Vert. Segments", "-", "Orientation", "Max Feret Diameter Orientation", "-", "% Area/Image Area", "% Area/(Particle & Holes' Area)", "Ratio of Equivalent Ellipse Axes", "Ratio of Equivalent Rect Sides", "-", "Elongation Factor", "Compactness Factor", "Heywood Circularity Factor", "Type Factor", "-", "Sum X", "Sum Y", "Sum XX", "Sum XY", "Sum YY", "Sum XXX", "Sum XXY", "Sum XYY", "Sum YYY", "-", "Moment of Inertia XX", "Moment of Inertia XY", "Moment of Inertia YY", "Moment of Inertia XXX", "Moment of Inertia XXY", "Moment of Inertia XYY", "Moment of Inertia YYY", "Norm. Moment of Inertia XX", "Norm. Moment of Inertia XY", "Norm. Moment of Inertia YY", "Norm. Moment of Inertia XXX", "Norm. Moment of Inertia XXY", "Norm. Moment of Inertia XYY", "Norm. Moment of Inertia YYY", "Hu Moment 1", "Hu Moment 2", "Hu Moment 3", "Hu Moment 4", "Hu Moment 5", "Hu Moment 6", "Hu Moment 7"] ("Measurement Parameter")
              w323 = T2 0 items=["Center of Mass X", "Center of Mass Y", "First Pixel X", "First Pixel Y", "Bounding Rect Left", "Bounding Rect Top", "Bounding Rect Right", "Bounding Rect Bottom", "Max Feret Diameter Start X", "Max Feret Diameter Start Y", "Max Feret Diameter End X", "Max Feret Diameter End Y", "Max Horiz. Segment Length Left", "Max Horiz. Segment Length Right", "Max Horiz. Segment Length Row", "-", "Bounding Rect Width", "Bounding Rect Height", "Bounding Rect Diagonal", "Perimeter", "Convex Hull Perimeter", "Holes' Perimeter", "Max Feret Diameter", "Equivalent Ellipse Major Axis", "Equivalent Ellipse Minor Axis", "Equivalent Ellipse Minor Axis (Feret)", "Equivalent Rect Long Side", "Equivalent Rect Short Side", "Equivalent Rect Diagonal", "Equivalent Rect Short Side (Feret)", "Average Horiz. Segment Length", "Average Vert. Segment Length", "Hydraulic Radius", "Waddel Disk Diameter", "-", "Area", "Holes' Area", "Particle & Holes' Area", "Convex Hull Area", "Image Area", "-", "Number of Holes", "Number of Horiz. Segments", "Number of Vert. Segments", "-", "Orientation", "Max Feret Diameter Orientation", "-", "% Area/Image Area", "% Area/(Particle & Holes' Area)", "Ratio of Equivalent Ellipse Axes", "Ratio of Equivalent Rect Sides", "-", "Elongation Factor", "Compactness Factor", "Heywood Circularity Factor", "Type Factor", "-", "Sum X", "Sum Y", "Sum XX", "Sum XY", "Sum YY", "Sum XXX", "Sum XXY", "Sum XYY", "Sum YYY", "-", "Moment of Inertia XX", "Moment of Inertia XY", "Moment of Inertia YY", "Moment of Inertia XXX", "Moment of Inertia XXY", "Moment of Inertia XYY", "Moment of Inertia YYY", "Norm. Moment of Inertia XX", "Norm. Moment of Inertia XY", "Norm. Moment of Inertia YY", "Norm. Moment of Inertia XXX", "Norm. Moment of Inertia XXY", "Norm. Moment of Inertia XYY", "Norm. Moment of Inertia YYY", "Hu Moment 1", "Hu Moment 2", "Hu Moment 3", "Hu Moment 4", "Hu Moment 5", "Hu Moment 6", "Hu Moment 7"] ("Measurement Parameter")
              w326 = T5 0 items=["Grayscale (U8)", "Grayscale (I16)", "Grayscale (SGL)", "Complex (CSG)", "RGB (U32)", "HSL (U32)", "RGB (U64)", "Grayscale (U16)"] ("Image Type")
              n146 = Add(x=w301, y=2.0) -> (x+y=w305:dbl)
              n147 = Subtract(x=w301, y=2.0) -> (x-y=w299:dbl)
              n148 = Bundle("Measurement Parameter"=w323, w299, w305, "Range"=FALSE, "Measurement Type"=FALSE) -> (w317:T7)  [unwired: 1 out]
              n149 = call "IMAQ Create"("Image Name"="17", "Image Type"=w303) -> ("New Image"=w302:T1)  [unwired: 2 in, 2 out]
              n150 = Add(x=w295, y=2.0) -> (x+y=w293:dbl)
              n151 = Subtract(x=w295, y=2.0) -> (x-y=w294:dbl)
              n152 = Bundle("Measurement Parameter"=w320, w294, w293, "Range"=FALSE, "Measurement Type"=FALSE) -> (w292:T7)  [unwired: 1 out]
              n153 = Build Array(w317) -> (w298:T8)
              n154 = Build Array(w292) -> (w291:T8)
              n155 = Number To Decimal String(number=w313) -> (decimal integer string=w312:string)  [unwired: 1 out]
              n156 = call "IMAQ Particle Filter 3"("Image Src"=w324, "Image Dst"=w302, "Selection Values"=w298, "Keep/Remove Particles (F)"=FALSE) -> ("Image Dst Out"=w310:T1)  [unwired: 5 in, 6 out]
              n157 = Subtract(x=180.0, y=w316) -> (x-y=w314:dbl)
              n158 = call "IMAQ Create"("Image Name"="16", "Image Type"=w326) -> ("New Image"=w308:T1)  [unwired: 2 in, 2 out]
              n159 = call "IMAQ Particle Filter 3"("Image Src"=w310, "Image Dst"=w308, "Selection Values"=w291, "Keep/Remove Particles (F)"=FALSE) -> ("Image Dst Out"=w285:T1, "Number of Particles"=w307:i32)  [unwired: 5 in, 5 out]
              n160 = call "IMAQ Create"("Image Name"="18", "Image Type"=w290) -> ("New Image"=w288:T1)  [unwired: 2 in, 2 out]
              n161 = call "IMAQ Rotate"("Maintain Size"=FALSE, "Angle (degrees)"=w314, "Image Dst"=w288, "Image Src"=w285) -> ("Image Dst Out"=w283:T1)  [unwired: 4 in, 3 out]
              "属于某个角度下图像" <- w283
              n162 = disable-structure shown="Enabled" {
                disable-tunnel: w312 -> [w335 _]
                disable-tunnel: w283 -> [w327 _]
                frame Disabled {
                  n163 = Current VI's Path() -> (path=w328:path)
                  n164 = Strip Path(path=w328) -> (stripped path=w331:path)  [unwired: 1 out]
                  n165 = Concatenate Strings("2" ("string"), "-" ("string"), w335, ".png") -> (w332:string)
                  n166 = Build Path(base path=w331, name or relative path=w332) -> (appended path=w330:path)
                  n167 = call-poly "IMAQ Write File 2"("File Path"=w330, "Image"=w327) -> ()  [unwired: 4 in, 6 out]
                }
                frame Enabled {
                }
              }
              n168 = call "IMAQ Particle Analysis"("Pixel Measurements"=w287, "Image"=w283) -> ("Particle Measurements (Pixels)"=w284:dbl[][])  [unwired: 3 in, 6 out]
              n169 = call "IMAQ Particle Analysis"("Pixel Measurements"=w282, "Image"=w283) -> ("Particle Measurements (Pixels)"=w281:dbl[][])  [unwired: 3 in, 6 out]
            }
            n170 = for {
              tunnel: w257 -> [w280] mode=indexing
              tunnel: [w279] -> w260 mode=indexing
              n171 = Index Array(array=w280) -> (element=w279:dbl[])  [unwired: 2 in]
            }
            n172 = for {
              tunnel: w258 -> [w276] mode=indexing
              tunnel: [w275] -> w259 mode=indexing
              n173 = Index Array(array=w276) -> (element=w275:dbl[])  [unwired: 2 in]
            }
            n174 = for {
              tunnel: w260 -> [w278] mode=indexing
              tunnel: [w277] -> w256 mode=indexing
              n175 = Index Array(array=w278) -> (element=w277:dbl)  [unwired: 1 in]
            }
            "粒长" <- w256
            n176 = for {
              tunnel: w259 -> [w274] mode=indexing
              tunnel: [w273] -> w255 mode=indexing
              n177 = Index Array(array=w274) -> (element=w273:dbl)  [unwired: 1 in]
            }
            "粒宽" <- w255
            n178 = call <vilib>:"Std Deviation and Variance.vi"("X"=w256) -> ("mean"=w253:dbl, "standard deviation"=w252:dbl)  [unwired: 1 in, 1 out]
            "mean 2" <- w253
            "standard deviation 2" <- w252
            n179 = call <vilib>:"Std Deviation and Variance.vi"("X"=w255) -> ("mean"=w251:dbl, "standard deviation"=w250:dbl)  [unwired: 1 in, 1 out]
            "mean 3" <- w251
            "standard deviation 3" <- w250
            n180 = Divide(x=w256, y=w255) -> (x/y=w254:dbl[])
            "长宽比" <- w254
            n181 = call <vilib>:"Std Deviation and Variance.vi"("X"=w254) -> ("mean"=w249:dbl, "standard deviation"=w248:dbl)  [unwired: 1 in, 1 out]
            "mean 4" <- w249
            "standard deviation 4" <- w248
          }
          frame #2 {
            n182 = Tick Count (ms)() -> (millisecond timer value=w344:u32)
            n183 = Subtract(x=w344, y=w343) -> (x-y=→"耗时":u32)
          }
        }
        n184 = call "IMAQ Particle Analysis"("Pixel Measurements"=w169, "Image"=w167) -> ("Particle Measurements (Pixels)"=w161:dbl[][])  [unwired: 3 in, 6 out]
        n185 = Index Array(array=w161, index (col)=0 ("index (row)")) -> (element=w160:dbl[])  [unwired: 1 in]
        "Area" <- w160
        n186 = Index Array(array=w161, index (col)=1 ("index (row)")) -> (element=w159:dbl[])  [unwired: 1 in]
        "Perimeter" <- w159
        n187 = Index Array(array=w161, index (col)=2 ("index (row)")) -> (element=w158:dbl[])  [unwired: 1 in]
        "AR" <- w158
        n188 = Index Array(array=w161, index (col)=3 ("index (row)")) -> (element=w157:dbl[])  [unwired: 1 in]
        "Equivalent ellipse" <- w157
        n189 = Index Array(array=w161, index (col)=4 ("index (row)")) -> (element=w156:dbl[])  [unwired: 1 in]
        "Circularity" <- w156
        n190 = call <vilib>:"Std Deviation and Variance.vi"("X"=w160) -> ("mean"=w146:dbl, "standard deviation"=w145:dbl)  [unwired: 1 in, 1 out]
        "mean 5" <- w146
        "standard deviation 5" <- w145
        n191 = call <vilib>:"Std Deviation and Variance.vi"("X"=w158) -> ("mean"=w142:dbl, "standard deviation"=w141:dbl)  [unwired: 1 in, 1 out]
        "mean 7" <- w142
        "standard deviation 7" <- w141
        n192 = call <vilib>:"Std Deviation and Variance.vi"("X"=w157) -> ("mean"=w140:dbl, "standard deviation"=w139:dbl)  [unwired: 1 in, 1 out]
        "mean 8" <- w140
        "standard deviation 8" <- w139
        n193 = call <vilib>:"Std Deviation and Variance.vi"("X"=w159) -> ("mean"=w144:dbl, "standard deviation"=w143:dbl)  [unwired: 1 in, 1 out]
        "mean 6" <- w144
        "standard deviation 6" <- w143
        n194 = call <vilib>:"Std Deviation and Variance.vi"("X"=w156) -> ("mean"=w138:dbl, "standard deviation"=w137:dbl)  [unwired: 1 in, 1 out]
        "mean 9" <- w138
        "standard deviation 9" <- w137
        n195 = Build Array(w154, w153, w152, w151, w150, w149, w146, w145, w144, w143, w142, w141, w140, w139, w138, w137) -> (w148:dbl[])
        n196 = Number To Fractional String(number=w148) -> (F-format string=w147:string[])  [unwired: 3 in]
        n197 = Number To Decimal String(number=w194) -> (decimal integer string=w193:string)  [unwired: 1 in]
        n198 = Build Array (concatenate)(w195, w193, w147) -> (w192:string[])
        n199 = call-poly <vilib>:"Write Delimited Spreadsheet.vi"("file path (dialog if empty)"="数据存储", "1D data"=w192, "append to file? (new file:F)"=TRUE ("append to file? (F)")) -> ()  [unwired: 11 in, 2 out]
      }
    }
    n200 = local read "Path(part2)"() -> (w10:path)
    n201 = local read "Path(part1)"() -> (w9:path)
    n202 = Build Array(w10, w9) -> (w8:path[])
    n203 = for {
      tunnel: [w27] -> w13 mode=indexing
      tunnel: w8 -> [w26] mode=indexing
      n204 = Strip Path(path=w26) -> (stripped path=w29:path, name=w30:string)
      n205 = String Subset(string=w30, offset (0)=2, length (rest)=1 ("length (rest)")) -> (substring=w32:string)
      n206 = Equal?(x=w32, y="-") -> (x = y?=w28:bool)
      n207 = case shown="False" w28 {
        tunnel: w30 -> [w38 w84]
        tunnel: w30 -> [w37 w83]
        tunnel: w29 -> [w36 w85]
        tunnel: [w35 w82] -> w27
        frame False {
          n208 = Decimal String To Number(string=w38, offset=5) -> (number=w42:i32)  [unwired: 1 in, 1 out]
          n209 = Equal?(x=w42, y=5) -> (x = y?=w41:bool)
          n210 = case shown="True" w41 {
            tunnel: w37 -> [w49 w66]
            tunnel: w36 -> [w43 w81]
            tunnel: [w44 w67] -> w35
            frame False {
              w51 = "p" ("string")
              n211 = String Subset(string=w49, offset (0)=5, length (rest)=1 ("length (rest)")) -> (substring=w46:string)
              n212 = Decimal String To Number(string=w49, offset=5) -> (number=w50:i32)  [unwired: 1 in, 1 out]
              n213 = Concatenate Strings(w51, w46) -> (w52:string)
              n214 = Increment(x=w50) -> (x+1=w55:i32)
              n215 = Number To Decimal String(number=w55) -> (decimal integer string=w53:string)  [unwired: 1 in]
              n216 = Concatenate Strings(w51, w53) -> (w54:string)
              n217 = Search and Replace String(input string=w49, search string=w52, replace string=w54) -> (result string=w45:string)  [unwired: 5 in, 3 out]
              n218 = Build Path(base path=w43, name or relative path=w45) -> (appended path=w44:path)
            }
            frame True {
              w72 = "p" ("string")
              n219 = Strip Path(path=w81) -> (stripped path=w59:path, name=w80:string)
              n220 = String Subset(string=w66, offset (0)=5, length (rest)=1 ("length (rest)")) -> (substring=w75:string)
              n221 = Decimal String To Number(string=w80, offset=0) -> (number=w78:i32)  [unwired: 1 in, 1 out]
              n222 = String Subset(string=w66, offset (0)=4, length (rest)=8 ("length (rest)")) -> (substring=w65:string)
              n223 = Concatenate Strings(w72, w75) -> (w74:string)
              n224 = Concatenate Strings(w72, "1") -> (w71:string)
              n225 = Increment(x=w78) -> (x+1=w70:i32)
              n226 = Path To String(path=w59) -> (string=w61:string)
              n227 = Number To Decimal String(number=w70) -> (decimal integer string=w62:string)  [unwired: 1 in]
              n228 = Search and Replace String(input string=w65, search string=w74, replace string=w71) -> (result string=w58:string)  [unwired: 5 in, 3 out]
              n229 = Concatenate Strings(w61, "\\" ("string"), w62, "\\" ("string"), w62, "-", w58) -> (w68:string)
              n230 = String To Path(string=w68) -> (path=w67:path)
            }
          }
        }
        frame True {
          n231 = Decimal String To Number(string=w84, offset=4) -> (number=w89:i32)  [unwired: 1 in, 1 out]
          n232 = Equal?(x=w89, y=5) -> (x = y?=w88:bool)
          n233 = case shown="False" w88 {
            tunnel: w83 -> [w96 w113]
            tunnel: w85 -> [w90 w128]
            tunnel: [w91 w114] -> w82
            frame False {
              w98 = "p" ("string")
              n234 = String Subset(string=w96, offset (0)=4, length (rest)=1 ("length (rest)")) -> (substring=w93:string)
              n235 = Decimal String To Number(string=w96, offset=4) -> (number=w97:i32)  [unwired: 1 in, 1 out]
              n236 = Concatenate Strings(w98, w93) -> (w99:string)
              n237 = Increment(x=w97) -> (x+1=w102:i32)
              n238 = Number To Decimal String(number=w102) -> (decimal integer string=w100:string)  [unwired: 1 in]
              n239 = Concatenate Strings(w98, w100) -> (w101:string)
              n240 = Search and Replace String(input string=w96, search string=w99, replace string=w101) -> (result string=w92:string)  [unwired: 5 in, 3 out]
              n241 = Build Path(base path=w90, name or relative path=w92) -> (appended path=w91:path)
            }
            frame True {
              w119 = "p" ("string")
              n242 = Strip Path(path=w128) -> (stripped path=w106:path, name=w127:string)
              n243 = String Subset(string=w113, offset (0)=4, length (rest)=1 ("length (rest)")) -> (substring=w122:string)
              n244 = Decimal String To Number(string=w127, offset=0) -> (number=w125:i32)  [unwired: 1 in, 1 out]
              n245 = String Subset(string=w113, offset (0)=3, length (rest)=8 ("length (rest)")) -> (substring=w112:string)
              n246 = Concatenate Strings(w119, w122) -> (w121:string)
              n247 = Concatenate Strings(w119, "1") -> (w118:string)
              n248 = Increment(x=w125) -> (x+1=w117:i32)
              n249 = Path To String(path=w106) -> (string=w108:string)
              n250 = Number To Decimal String(number=w117) -> (decimal integer string=w109:string)  [unwired: 1 in]
              n251 = Search and Replace String(input string=w112, search string=w121, replace string=w118) -> (result string=w105:string)  [unwired: 5 in, 3 out]
              n252 = Concatenate Strings(w108, "\\" ("string"), w109, "\\" ("string"), w109, "-", w105) -> (w115:string)
              n253 = String To Path(string=w115) -> (path=w114:path)
            }
          }
        }
      }
    }
    n254 = Index Array(array=w13, index #1=0 ("index"), index #2=1 ("index")) -> (element #1=w12:path, element #2=w11:path)
    "Path(part2)" <- w24
    "Path(part1)" <- w16
    "Boolean" <- FALSE
  }
